vi "Read Actions.vi"(8 "error in (no error)":errorcluster, 11 "EventsAbstract in":refnum<class "EventsAbstract.lvclass">) -> (0 "error out":errorcluster, 2 "Actions":T1, 3 "EventsAbstract out":refnum<class "EventsAbstract.lvclass">)   [LabVIEW 2019, in "EventsAbstract.lvclass"]
uses:
  EventsAbstract.lvclass
  TypeDef/Event Actions.ctl
  Modules/ModuleAbstract/ModuleAbstract/TypeDef/Module Actions.ctl
  <vilib>/ActorFramework/Message Enqueuer/Message Enqueuer.lvclass
  EventsAbstract.lvclass/EventsAbstract.ctl
  Modules/ModuleAbstract/ModuleAbstract/ModuleAbstract.lvclass
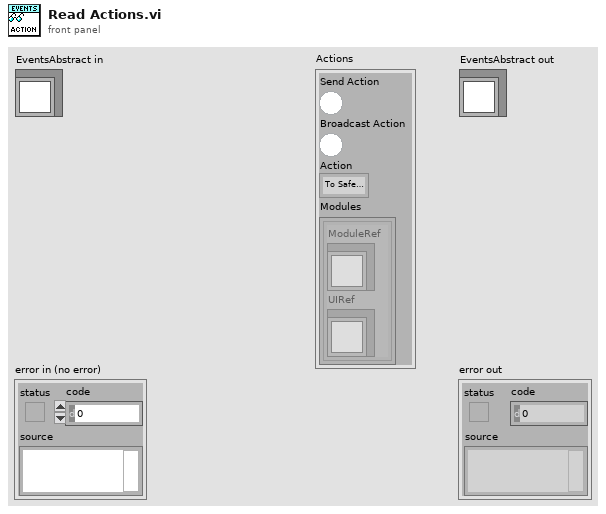
[diagram p1: front panel]
types:
  T1 = typedef "EventsAbstract.lvclass/Event Actions.ctl" = cluster{"Send Action":bool, "Broadcast Action":bool, "Action":T2, "Modules":cluster{"ModuleRef":refnum<class "Message Enqueuer.lvclass">, "UIRef":refnum<class "Message Enqueuer.lvclass">}[]}
  T2 = typedef "ModuleAbstract.lvlib/ModuleAbstract.lvclass/Module Actions.ctl" = enum16{"To Safe State", "Reset Safe State", "Close Module"}
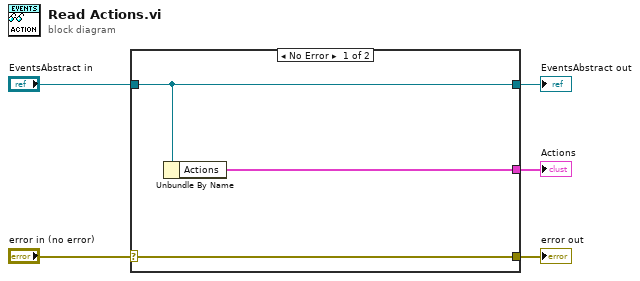
[diagram p0: block diagram]
diagram:
  n1 = case shown="No Error" "error in (no error)" {
    selector: "error in (no error)" -> [w8 w9]
    tunnel: [w8 w9] -> w4
    tunnel: [w7 w10] -> w2
    tunnel: "EventsAbstract in" -> [w7 w10]
    tunnel: [w6 _] -> w1
    frame No Error {
      n2 = Unbundle By Name(w7) -> ("Actions"=w6:T1)
    }
    frame Error {
    }
  }
  "error out" <- w4
  "EventsAbstract out" <- w2
  "Actions" <- w1
